vi "Save-Load Triggers Output Setup.vi"(6 "Which file? (User profile.ini)":T3=enum."Loaded User profile.ini", 8 "error in":errorcluster, 9 "General trigger settings":T1={"Trigger 1 function"=enum."Encoder trigger", "Triggers loop clock (MHz)"=80.0} {"Triggers loop clock (MHz)" format="%#_13g"}, 10 "Triggers output setup to save":T4=[{"Name"="Unused", "Output?"=FALSE, "Output terminal"="/PXI1Slot6/PFI0", "PXI backplane line"="/PXI1Slot6/PXI_Trig0", "Pulse width (us)"=20}, {"Name"="Line trigger", "Output?"=FALSE, "Output terminal"="/PXI1Slot6/PFI1", "PXI backplane line"="/PXI1Slot6/PXI_Trig1", "Pulse width (us)"=20}, {"Name"="Frame trigger / Trial trigger", "Output?"=FALSE, "Output terminal"="/PXI1Slot6/PFI2", "PXI backplane line"="/PXI1Slot6/PXI_Trig2", "Pulse width (us)"=20}, {"Name"="Cycle trigger", "Output?"=FALSE, "Output terminal"="/PXI1Slot6/PFI3", "PXI backplane line"="/PXI1Slot6/PXI_Trig3", "Pulse width (us)"=20}, {"Name"="Start of Experiment trigger", "Output?"=FALSE, "Output terminal"="/PXI1Slot6/PFI4", "PXI backplane line"="/PXI1Slot6/PXI_Trig4", "Pulse width (us)"=20}, {"Name"="Stimulus trigger", "Output?"=FALSE, "Output terminal"="/PXI1Slot6/PFI5", "PXI backplane line"="/PXI1Slot6/PXI_Trig5", "Pulse width (us)"=20}] {"Pulse width (us)" min=10 max=5000 step=1 format="%.0fµs"}, 11 "Function":T6=enum."Load from file") -> (0 "error out":errorcluster, 1 "General trigger settings":T1={"Trigger 1 function"=enum."Encoder trigger", "Triggers loop clock (MHz)"=80.0} {"Triggers loop clock (MHz)" format="%#_13g"}, 2 "Triggers output setup":T4=[{"Name"="", "Output?"=FALSE, "Output terminal"="/PXI1Slot6/PFI0", "PXI backplane line"="/PXI1Slot6/PXI_Trig0", "Pulse width (us)"=20}, {"Name"="", "Output?"=FALSE, "Output terminal"="/PXI1Slot6/PFI0", "PXI backplane line"="/PXI1Slot6/PXI_Trig0", "Pulse width (us)"=20}, {"Name"="", "Output?"=FALSE, "Output terminal"="/PXI1Slot6/PFI0", "PXI backplane line"="/PXI1Slot6/PXI_Trig0", "Pulse width (us)"=20}, {"Name"="", "Output?"=FALSE, "Output terminal"="/PXI1Slot6/PFI0", "PXI backplane line"="/PXI1Slot6/PXI_Trig0", "Pulse width (us)"=20}, {"Name"="", "Output?"=FALSE, "Output terminal"="/PXI1Slot6/PFI0", "PXI backplane line"="/PXI1Slot6/PXI_Trig0", "Pulse width (us)"=20}, {"Name"="", "Output?"=FALSE, "Output terminal"="/PXI1Slot6/PFI0", "PXI backplane line"="/PXI1Slot6/PXI_Trig0", "Pulse width (us)"=20}] {"Pulse width (us)" min=10 max=5000 step=1 format="%.0fµs"})   [LabVIEW 2020]
uses:
  Typedefs/Save-Load enum.ctl
  Peripherals Control/Triggers/Typedefs/Triggers output setup.ctl
  Peripherals Control/Triggers/Typedefs/Trigger setup element cluster.ctl
  Typedefs/Which path.ctl
  Peripherals Control/Triggers/Typedefs/General trigger settings cluster.ctl
  Typedefs/Trigger 1 selector enum.ctl
  <vilib>/Utility/config.llb/NI_LVConfig.lvlib
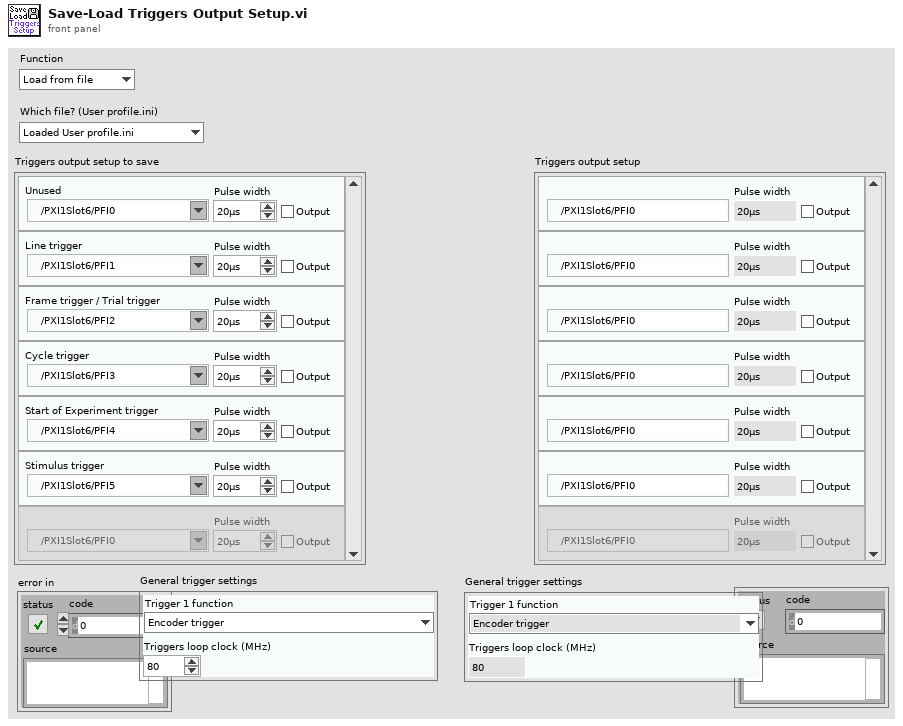
[diagram p1: front panel]
types:
  T1 = typedef "General trigger settings cluster.ctl" = cluster{"Trigger 1 function":T2, "Triggers loop clock (MHz)":dbl}
  T2 = typedef "Trigger 1 selector enum.ctl" = enum16{"Encoder trigger", "Line trigger", "Control system's ref frame acknowledgement"}
  T3 = typedef "Which path.ctl" = enum16{"Configuration Files", "Calibration Files", "Images", "Setup.ini", "Loaded User profile.ini", "User's-Previous session.ini", "New user profile.ini", "Selected User profile.ini", "User profiles folder", "Power meter scaling.txt", "FOV Cal.ini", "Calibration.ini"}
  T4 = typedef "Triggers output setup.ctl" = T5[]
  T5 = typedef "Trigger setup element cluster.ctl" = cluster{"Name":string, "Output?":bool, "Output terminal":tag, "PXI backplane line":tag, "Pulse width (us)":u16}
  T6 = typedef "Save-Load enum.ctl" = enum16{"Save to file", "Load from file", "Compare from file", "Save Backup"}
  T7 = typedef "NI_LVConfig.lvlib/Config Data RefNum.ctl" = refnum<k1>
  T8 = typedef "Ini file interface (String).ctl" = cluster{"key":string, "Save?":bool, "Default":string}[]
  T9 = typedef "Ini file interface (DBL).ctl" = cluster{"key":string, "Save?":bool, "Default":dbl}[]
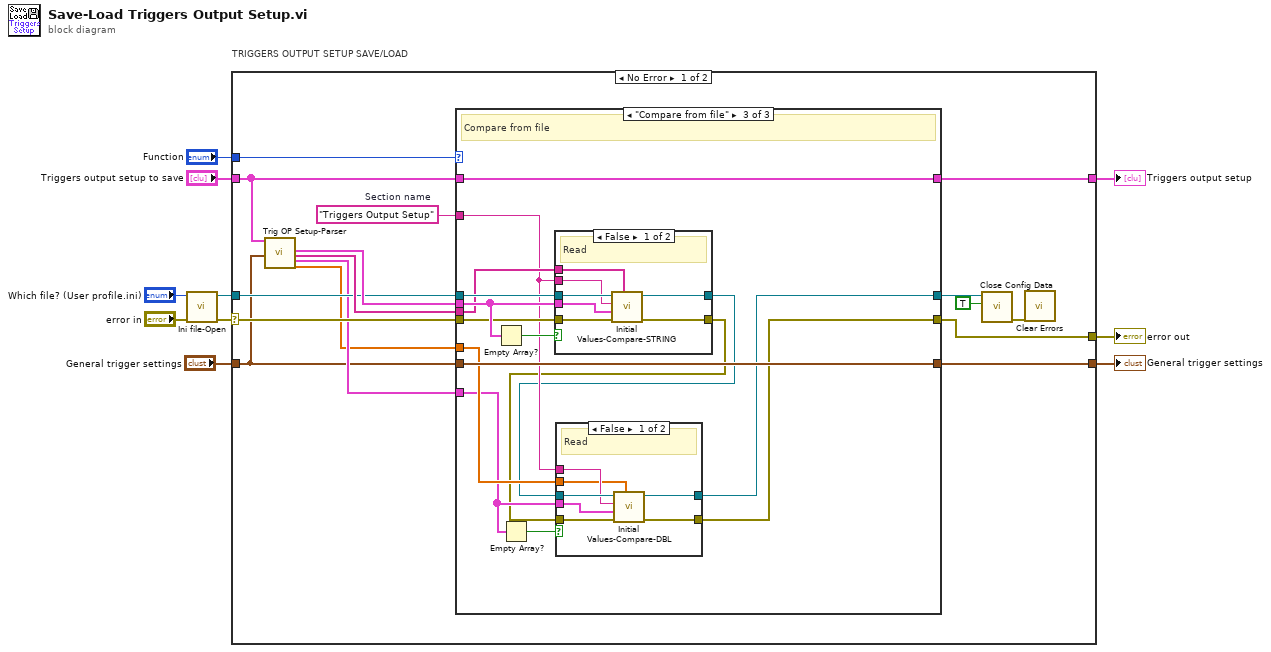
[diagram p0: block diagram]
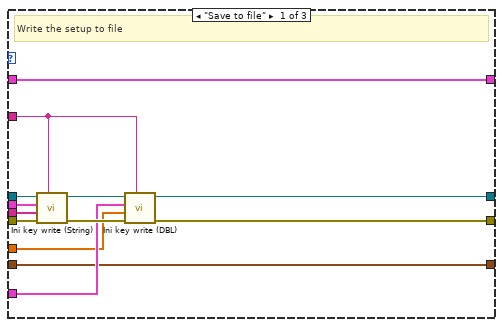
[diagram p2: hidden frame]
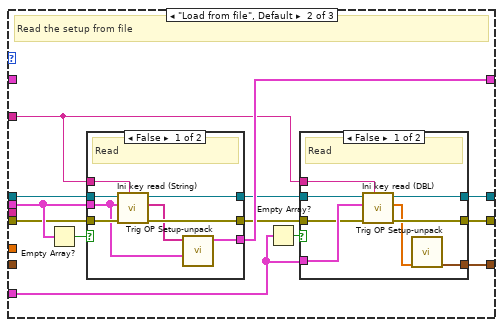
[diagram p3: hidden frame]
diagram:
  n1 = call "Ini file-Open.vi"("Error In"="error in", "Which file?"="Which file? (User profile.ini)") -> ("error out"=w9:errorcluster, "User profile ini file ref"=w7:T7)  [unwired: 6 in, 2 out]
  n2 = case "TRIGGERS OUTPUT SETUP SAVE/LOAD" shown="No Error" w9 {
    selector: w9 -> [w17 w108]
    tunnel: [w15 w108] -> w6
    tunnel: "Triggers output setup to save" -> [w21 w107]
    tunnel: [w22 w107] -> w4
    tunnel: "Function" -> [w18 _]
    tunnel: w7 -> [w16 _]
    tunnel: "General trigger settings" -> [w11 w106]
    tunnel: [w12 w106] -> w1
    frame No Error {
      w26 = "Triggers Output Setup"  # Section name
      n3 = call "Trig OP Setup-Parser.vi"("Triggers output setup to save"=w21, "General trigger settings"=w11) -> ("Keys setup.Strings"=w20:T8, "Values.Strings"=w19:string[], "Keys setup.DBL"=w14:T9, "Values.DBL"=w13:dbl[])  [unwired: 14 in]
      n4 = case shown="\"Compare from file\"" w18 {
        tunnel: [w30 w45 w73] -> w15
        tunnel: [w32 w46 w75] -> w24
        tunnel: w17 -> [w35 w50 w85]
        tunnel: w16 -> [w36 w49 w84]
        tunnel: w26 -> [w34 w42 w77]
        tunnel: w19 -> [w38 _ w82]
        tunnel: w20 -> [w39 w51 w86]
        tunnel: [w37 w48 w83] -> w22
        tunnel: w21 -> [w37 _ w83]
        tunnel: w14 -> [w29 w40 w79]
        tunnel: w13 -> [w28 _ w80]
        tunnel: w11 -> [w27 _ w81]
        tunnel: [w27 w43 w81] -> w12
        frame "Save to file" {
          # "Write the setup to file"
          n5 = call "Ini key write (String).vi"("Section"=w34, "error in (no error)"=w35, "Values (String)"=w38, "Ini file interface"=w39, "Ini file refnum in"=w36) -> ("error out"=w31:errorcluster, "Ini file refnum out"=w33:T7)  [unwired: 5 in]
          n6 = call "Ini key write (DBL).vi"("Section"=w34, "error in (no error)"=w31, "Values (DBL)"=w28, "Ini file interface"=w29, "Ini file refnum in"=w33) -> ("error out"=w30:errorcluster, "Ini file refnum out"=w32:T7)  [unwired: 5 in]
        }
        frame "Load from file", Default {
          # "Read the setup from file"
          n7 = Empty Array?(array=w51) -> (empty?=w52:bool)
          n8 = case shown="False" w52 {
            tunnel: [w69 w72] -> w47
            tunnel: [w68 w71] -> w44
            tunnel: w51 -> [w64 _]
            tunnel: w49 -> [w70 w72]
            tunnel: w50 -> [w67 w71]
            tunnel: w42 -> [w63 _]
            tunnel: [w66 _] -> w48
            frame False {
              # "Read"
              n9 = call "Ini key read (String).vi"("Section name"=w63, "error in (no error)"=w67, "Keys setup"=w64, "Ini file ref in"=w70) -> ("error out"=w68:errorcluster, "Value read/used"=w65:string[], "Ini file ref"=w69:T7)  [unwired: 5 in]
              n10 = call "Trig OP Setup-unpack.vi"("Keys setup"=w64, "Value read/used"=w65) -> ("Triggers output setup"=w66:T4)  [unwired: 8 in, 1 out]
            }
            frame True {
              # "Empty setup"
            }
          }
          n11 = Empty Array?(array=w40) -> (empty?=w41:bool)
          n12 = case shown="False" w41 {
            tunnel: [w59 w62] -> w46
            tunnel: [w56 w61] -> w45
            tunnel: w47 -> [w60 w62]
            tunnel: w44 -> [w57 w61]
            tunnel: w40 -> [w58 _]
            tunnel: w42 -> [w55 _]
            tunnel: [w53 _] -> w43
            frame False {
              # "Read"
              n13 = call "Ini key read (DBL).vi"("Section name"=w55, "error in (no error)"=w57, "Parameter names & setup"=w58, "Ini file refnum in"=w60) -> ("error out"=w56:errorcluster, "Value read/used"=w54:dbl[], "Ini file refnum out"=w59:T7)  [unwired: 5 in]
              n14 = call "Trig OP Setup-unpack.vi"("Values"=w54) -> ("output cluster"=w53:T1)  [unwired: 9 in, 1 out]
            }
            frame True {
              # "Empty setup"
            }
          }
        }
        frame "Compare from file" {
          # "Compare from file"
          n15 = Empty Array?(array=w86) -> (empty?=w87:bool)
          n16 = Empty Array?(array=w79) -> (empty?=w78:bool)
          n17 = case shown="False" w87 {
            tunnel: [w102 w105] -> w76
            tunnel: [w97 w104] -> w74
            tunnel: w86 -> [w100 _]
            tunnel: w84 -> [w103 w105]
            tunnel: w85 -> [w98 w104]
            tunnel: w77 -> [w101 _]
            tunnel: w82 -> [w99 _]
            frame False {
              # "Read"
              n18 = call "Initial Values-Compare-STRING.vi"("Current values"=w99, "error in (no error)"=w98, "Keys Array"=w100, "Section name"=w101, "User profile ini file ref"=w103) -> ("error out"=w97:errorcluster, "User profile ini file ref"=w102:T7)  [unwired: 2 in, 3 out]
            }
            frame True {
              # "Empty setup"
            }
          }
          n19 = case shown="False" w78 {
            tunnel: w76 -> [w94 w96]
            tunnel: [w93 w96] -> w75
            tunnel: [w92 w95] -> w73
            tunnel: w74 -> [w91 w95]
            tunnel: w77 -> [w89 _]
            tunnel: w79 -> [w90 _]
            tunnel: w80 -> [w88 _]
            frame False {
              # "Read"
              n20 = call "Initial Values-Compare-DBL.vi"("Current values"=w88, "error in (no error)"=w91, "Keys Array"=w90, "Section name"=w89, "User profile ini file ref"=w94) -> ("error out"=w92:errorcluster, "User profile ini file ref"=w93:T7)  [unwired: 2 in, 3 out]
            }
            frame True {
              # "No parametersof such type"
            }
          }
        }
      }
      n21 = call <vilib>:"Close Config Data.vi"("write file if changed (T)"=TRUE ("write configuration file? (F)"), "refnum"=w24) -> ("error out"=w23:errorcluster)  [unwired: 8 in, 1 out]
      n22 = call <vilib>:"Clear Errors.vi"("error in (no error)"=w23) -> ()  [unwired: 5 in, 2 out]
    }
    frame Error {
    }
  }
  "error out" <- w6
  "Triggers output setup" <- w4
  "General trigger settings" <- w1
